vi "Check and validate command.vi"(9 "Coherent laser commands L1":T2(ring), 10 "Commands & Queries":T5, 11 "Coherent Commands list":T3) -> (1 "Command String":string, 2 "Command Syntax":T7, 3 "Command validated ?":bool, 4 "Data Type":T1)   [LabVIEW 2020]
uses:
  Type defs/Command syntax.ctl
  Type defs/Commands List.ctl
  Type defs/coherent commands list.ctl
  Type defs/coherent commands.ctl
  Type defs/Command mode.ctl
  Type defs/data type.ctl
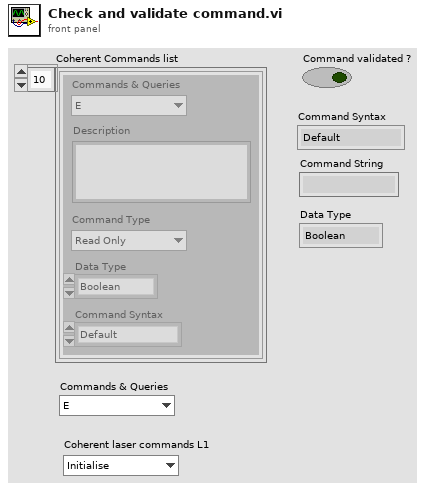
[diagram p1: front panel]
types:
  T1 = typedef "data type.ctl" = enum16{"Boolean", "Flag", "Numeric", "String", "Array"}
  T2 = enum16{"Initialise", "Get Command", "Set Command", "Close"}
  T3 = typedef "coherent commands list.ctl" = T4[]
  T4 = typedef "coherent commands.ctl" = cluster{"Description":string, "Commands & Queries":T5, "Command Type":T6, "Data Type":T1, "Command Syntax":T7}
  T5 = typedef "Commands List.ctl" = enum16{"E", "B", "FL", "HM", "L", "LBOH", "LBOOPT", "LFP", "PROMPT", "SM", "S", "VW", "VWS", "HB", "HBR", "REQ", "ALIGN", "K", "F", "FH", "UF", "PHLDC", "PZTMC", "PZTXC", "PZTYC", "PHLDP", "PZTMP", "PZTXP", "PZTYP", "PTRK", "MDLK", "PP", "TS", "STPRPOS", "C", "D1C", "D2C", "BT", "D1T", "D2T", "VT", "LBOT", "ET", "D1ST", "D2ST", "VST", "LBOST", "EST", "D1TD", "D2TD", "VD", "LBOD", "ED", "D1HST", "D2HST", "LRS", "D1SS", "D2SS", "VSS", "LBOSS", "ESS", "D1H", "D2H", "HH", "D1V", "D2V", "SV", "MB", "PI", "BV", "AMDLK", "PZTS", "TMAX", "TMIN", "ALIGNP", "ALIGNW", "PZTXCM", "PZTXCP", "PZTXPM", "PZTXPP", "PZTYCM", "PZTYCP", "PZTYPM", "PZTYPP", "RH", "SN", "ST", "GDDCURVE", "GDD", "GDDCURVEN", "SETCURVEN", "SETCURVEPT", "SAVECURVE", "DELCURVE", "CURVEN", "CURVEPT", "CURVE", "COMP", "HMCOMP", "GDDMAX", "GDDMIN"}
  T6 = typedef "Command mode.ctl" = enum16{"Read Only", "Write Only", "Read & Write"}
  T7 = typedef "Command syntax.ctl" = enum16{"Default", "Special"}
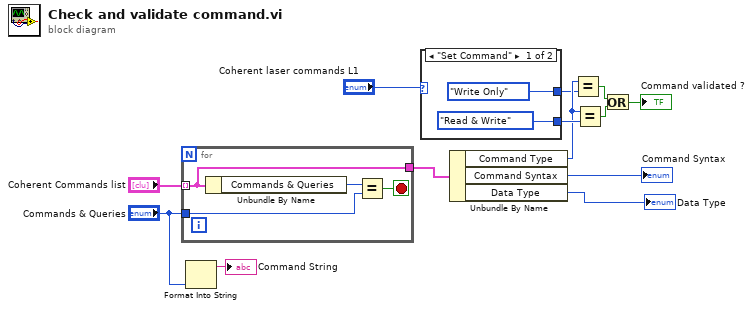
[diagram p0: block diagram]
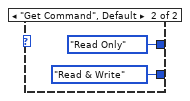
[diagram p2: hidden frame]
diagram:
  n1 = for {
    tunnel: "Coherent Commands list" -> [w15] mode=indexing
    tunnel: "Commands & Queries" -> [w14]
    tunnel: [w15] -> w6
    stop <- w16 stop-if-true
    n2 = Unbundle By Name(w15) -> ("Commands & Queries"=w17:T5)
    n3 = Equal?(x=w17, y=w14) -> (x = y?=w16:bool)
  }
  n4 = Format Into String("Commands & Queries") -> (resulting string=→"Command String":string)  [unwired: 3 in, 1 out]
  n5 = case shown="\"Set Command\"" "Coherent laser commands L1" {
    tunnel: [Command_mode."Read & Write" ("y") Command_mode."Read & Write" ("y")] -> w9
    tunnel: [Command_mode."Write Only" ("y") Command_mode."Read Only" ("y")] -> w7
    frame "Set Command" {
    }
    frame "Get Command", Default {
    }
  }
  n6 = Unbundle By Name(w6) -> ("Command Type"=w8:T6, "Command Syntax"=→"Command Syntax":T7, "Data Type"=→"Data Type":T1)
  n7 = Equal?(x=w8, y=w7) -> (x = y?=w10:bool)
  n8 = Equal?(x=w8, y=w9) -> (x = y?=w11:bool)
  n9 = Or(x=w10, y=w11) -> (x .or. y?=→"Command validated ?":bool)
